vi "Set VI Properties for Debugging Mode.vi"(6 "Red?":bool, 8 "error in":errorcluster, 10 "Debug mode?":bool, 11 "Launcher VI ref":refnum<vi>) -> (0 "error out":errorcluster, 3 "Launcher VI ref out":refnum<vi>)   [LabVIEW 2024, in "Launcher Support.lvlib"]
doc: "This VI sets the properties of the VI Launcher to either headless or debugging mode.\n_____\nBased on DQMH Dev Tools: Project Template 7.1.0.1503."
uses:
  Launcher Support.lvlib
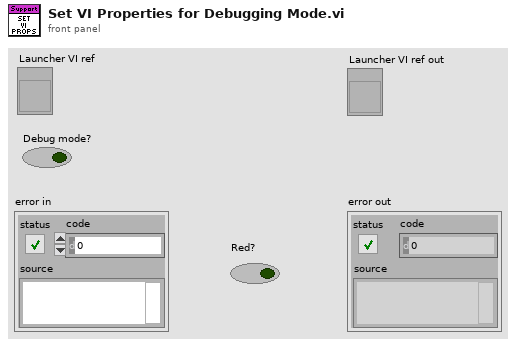
[diagram p1: front panel]
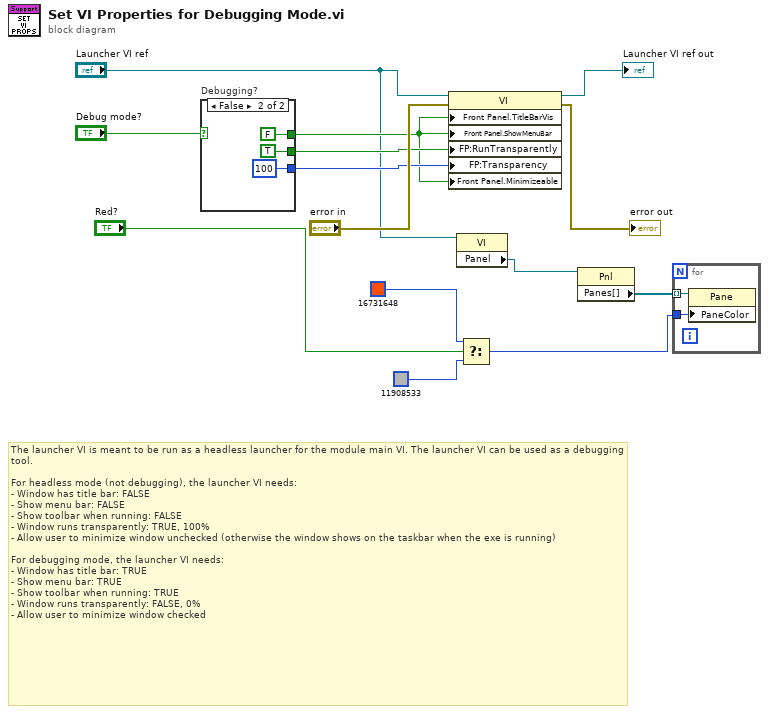
[diagram p0: block diagram]
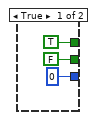
[diagram p2: hidden frame]
diagram:
  # "The launcher VI is meant to be run as a headless launcher for the module main VI. The launcher VI can be used as a debugging tool.\n\nFor headless mode (not debugging), the launcher VI needs:\n- Window has title bar: FALSE\n- Show menu bar: FALSE\n- Show toolbar when running: FALSE\n- Window runs transparently: TRUE, 100%\n- Allow user to minimize window unchecked (otherwise the window shows on the taskbar when the exe is running)\n\nFor debugging mode, the launcher VI needs:\n- Window has title bar: TRUE\n- Show menu bar: TRUE\n- Show toolbar when running: TRUE\n- Window runs transparently: FALSE, 0%\n- Allow user to minimize window checked"
  n1 = case "Debugging?" shown="False" "Debug mode?" {
    tunnel: [TRUE FALSE] -> w11
    tunnel: [FALSE TRUE] -> w13
    tunnel: [u8 0 ("Front Panel Window:Transparency") u8 100 ("Front Panel Window:Transparency")] -> w12
    frame True {
    }
    frame False {
    }
  }
  n2 = property class="VI"(reference="Launcher VI ref", error in="error in", "Front Panel.TitleBarVis"=w11, "Front Panel.ShowMenuBar"=w11, "FP:RunTransparently"=w13, "FP:Transparency"=w12, "Front Panel.Minimizeable"=w11) -> (reference out=→"Launcher VI ref out":refnum<vi>, error out=→"error out":errorcluster)
  n3 = property class="VI"(reference="Launcher VI ref") -> ("Panel"=w6:refnum<vi>)  [unwired: 1 in, 2 out]
  n4 = Select(t=u32 16731648, s="Red?", f=u32 11908533) -> (s? t:f=w2:u32)
  n5 = property class="Pnl"(reference=w6) -> ("Panes[]"=w5:refnum<vi>[])  [unwired: 1 in, 2 out]
  n6 = for {
    tunnel: w5 -> [w22] mode=indexing
    tunnel: w2 -> [w21]
    n7 = property class="Pane"(reference=w22, "PaneColor"=w21) -> ()  [unwired: 1 in, 2 out]
  }
